vi "serialRead.vi"(8 "error in (no error)":errorcluster, 11 "Python":T1) -> (0 "error out":errorcluster, 2 "Reply":string, 3 "Python out":T1)   [LabVIEW 2022 SP3]
uses:
  PythonCtrl.ctl
  Processors.ctl
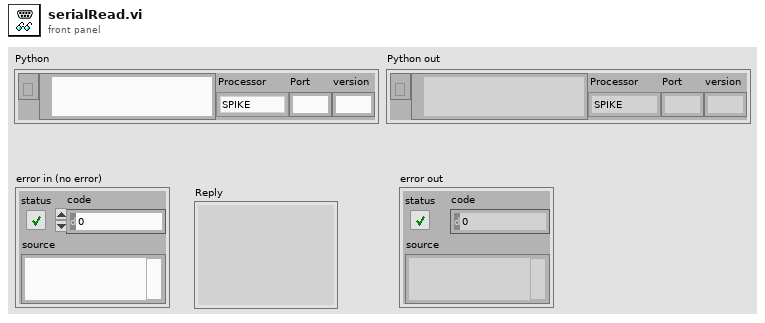
[diagram p1: front panel]
types:
  T1 = typedef "PythonCtrl.ctl" = cluster{"session":refnum<k35>, "PyPath":path, "Processor":T2, "Port":string, "version":string}
  T2 = typedef "Processors.ctl" = enum16{"SPIKE", "Pi", "Pi_ssh", "OpenMV", "Dunio"}
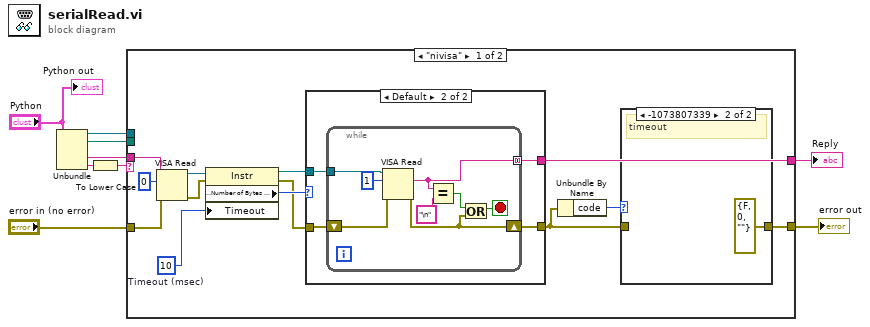
[diagram p0: block diagram]
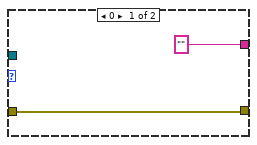
[diagram p3: hidden frame]
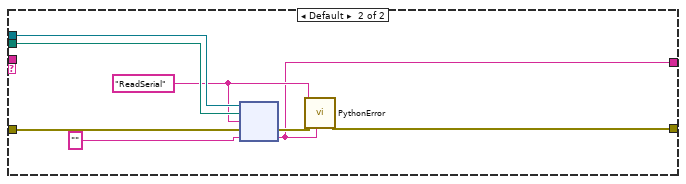
[diagram p4: hidden frame]
diagram:
  n1 = Unbundle("Python") -> ("session"=w8:refnum<k35>, "PyPath"=w9:path, "Port"=w2:string, "version"=w4:string)  [unwired: 1 out]
  n2 = To Lower Case(string=w4) -> (all lower case string=w3:string)
  n3 = case shown="\"nivisa\"" w3 {
    tunnel: w9 -> [_ w46]
    tunnel: w8 -> [_ w45]
    tunnel: "error in (no error)" -> [w16 w44]
    tunnel: [w12 w41] -> w5
    tunnel: w2 -> [w20 _]
    tunnel: [w22 w39] -> w1
    frame "nivisa" {
      w10 = u32 10  # Timeout (msec)
      n4 = VISA Read(VISA resource name=w20, byte count=u32 0, error in (no error)=w16) -> (VISA resource name out=w21:refnum<visa-resource-name>, error out=w17:errorcluster)  [unwired: 2 out]
      n5 = property class="Instr"(reference=w21, error in=w17, "Timeout"=w10) -> (reference out=w14:refnum<visa-resource-name>, error out=w15:errorcluster, "Serial Settings:Number of Bytes at Serial Port"=w18:u32)
      n6 = case shown="Default" w18 {
        tunnel: w14 -> [_ w30]
        tunnel: ["" ("read buffer") w29] -> w22
        tunnel: [w25 w28] -> w11
        tunnel: w15 -> [w25 w27]
        frame 0 {
        }
        frame Default {
          n7 = while {
            tunnel: w30 -> [w38]
            tunnel: [w36] -> w29 mode=concatenating
            shift-right: [w31] -> w28
            shift-left: w27 -> [w32]
            stop <- w33 stop-if-true
            n8 = VISA Read(VISA resource name=w38, byte count=u32 1, error in (no error)=w32) -> (read buffer=w36:string, error out=w31:errorcluster)  [unwired: 2 out]
            n9 = Equal?(x=w36, y="\n") -> (x = y?=w34:bool)
            n10 = Or(x=w34, y=w31) -> (x .or. y?=w33:bool)
          }
        }
      }
      n11 = Unbundle By Name(w11) -> ("code"=w13:i32)
      n12 = case shown="-1073807339" w13 {
        tunnel: [w23 errorcluster {"status"=FALSE, "code"=0, "source"=""} ("error out")] -> w12
        tunnel: w11 -> [w23 _]
        frame Default {
        }
        frame -1073807339 {
          # "timeout"
        }
      }
    }
    frame Default {
      w40 = "ReadSerial" ("function name")
      n13 = node(w45, w46, w40, w44, "" ("function name")) -> (w42:errorcluster, w39:string)  [unwired: 3 out]
      n14 = call "PythonError.vi"("reply"=w39, "error in (no error)"=w42, "function name"=w40) -> ("error out"=w41:errorcluster)  [unwired: 8 in]
    }
  }
  "error out" <- w5
  "Reply" <- w1
  "Python out" <- "Python"
